vi "isSignal.vi"(0 "reference":refnum<class "CallEdge.lvclass">, 5 "error in (no error)":errorcluster) -> (14 "reference out":refnum<class "CallEdge.lvclass">, 15 "signal":bool, 19 "error out":errorcluster)   [LabVIEW 2012, in "CallEdge.lvclass"]
doc: "public boolean isSignal()"
uses:
  <resource>/Framework/Providers/Open_GDS/UML/CallEdge_class/CallEdge.lvclass
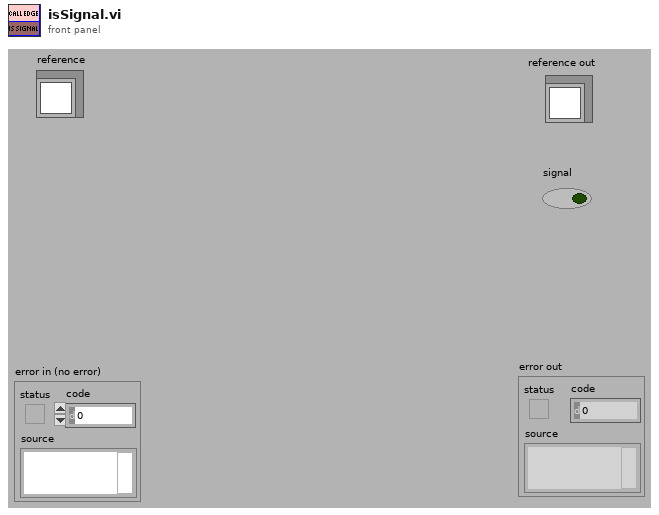
[diagram p1: front panel]
types:
  T1 = typedef "CallEdge.lvclass/ObjectAttributes.ctl" = cluster{"signal":bool}
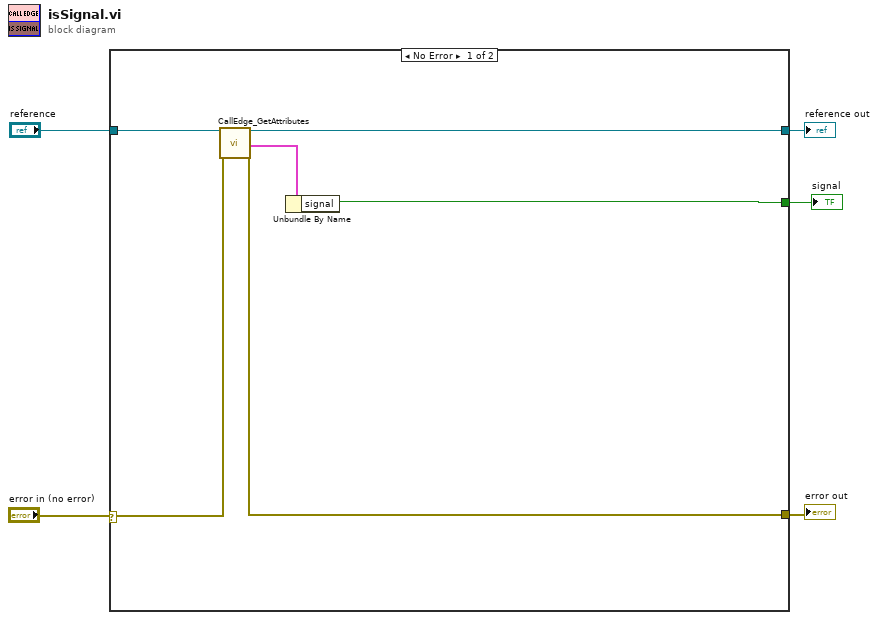
[diagram p0: block diagram]
diagram:
  n1 = case shown="No Error" "error in (no error)" {
    selector: "error in (no error)" -> [w8 w12]
    tunnel: "reference" -> [w11 w13]
    tunnel: [w10 w12] -> w4
    tunnel: [w9 w13] -> w3
    tunnel: [w7 _] -> w1
    frame No Error {
      n2 = call <resource>:"CallEdge_GetAttributes.vi"("reference in"=w11, "error in (no error)"=w8) -> ("reference out"=w9:refnum<class "CallEdge.lvclass">, "Data"=w6:T1, "error out"=w10:errorcluster)  [unwired: 1 in, 14 out]
      n3 = Unbundle By Name(w6) -> ("signal"=w7:bool)
    }
    frame Error {
    }
  }
  "reference out" <- w3
  "error out" <- w4
  "signal" <- w1
